vi "Ido_generalas.vi"(9 "Felbontas [s]":dbl=60.0, 10 "t_sim [nap]":dbl=7.0) -> (2 "t_vektor":dbl[](array[numeric]))   [LabVIEW 2013]
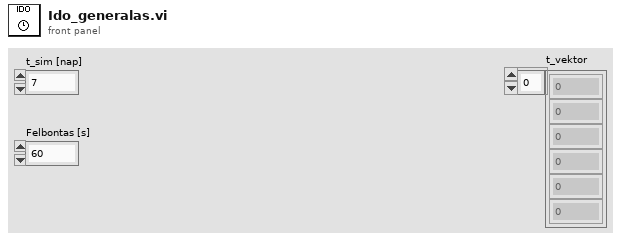
[diagram p1: front panel]
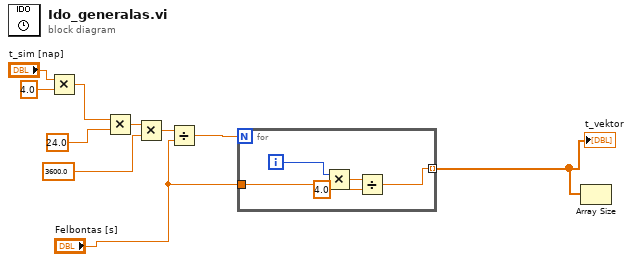
[diagram p0: block diagram]
diagram:
  n1 = Multiply(x="t_sim [nap]", y=4.0) -> (x*y=w2:dbl)
  n2 = Multiply(x=w2, y=24.0) -> (x*y=w9:dbl)
  n3 = Multiply(x=w9, y=3600.0) -> (x*y=w7:dbl)
  n4 = Divide(x=w7, y="Felbontas [s]") -> (x/y=w6:dbl)
  n5 = for {
    N: w6 -> [_]
    tunnel: [w11] -> w4 mode=indexing
    tunnel: "Felbontas [s]" -> [w14]
    i -> [w15]
    n6 = Multiply(x=w15, y=w14) -> (x*y=w13:dbl)
    n7 = Divide(x=w13, y=4.0) -> (x/y=w11:dbl)
  }
  "t_vektor" <- w4
  n8 = Array Size(array=w4) -> ()  [unwired: 1 out]
